vi "getConfigEventTest.vi"(8 "error in (no error)":errorcluster, 11 "SalProcess in":refnum<class "SalProcess.lvclass">) -> (0 "error out":errorcluster, 2 "configEventTest":cluster{"numOfTest":i32, "periodOfTestInMs":u32}, 3 "SalProcess out":refnum<class "SalProcess.lvclass">)   [LabVIEW 2018, in "SalProcess.lvclass"]
doc: "Get the configuration of event test."
uses:
  SalProcess.lvclass
  <vilib>/Utility/config.llb/Read Key (U32).vi
  <vilib>/Utility/config.llb/Read Key (I32).vi
  <vilib>/Utility/config.llb/NI_LVConfig.lvlib
panel:
  in  "configEventTestIn":cluster{"numOfTest":i32, "periodOfTestInMs":u32}
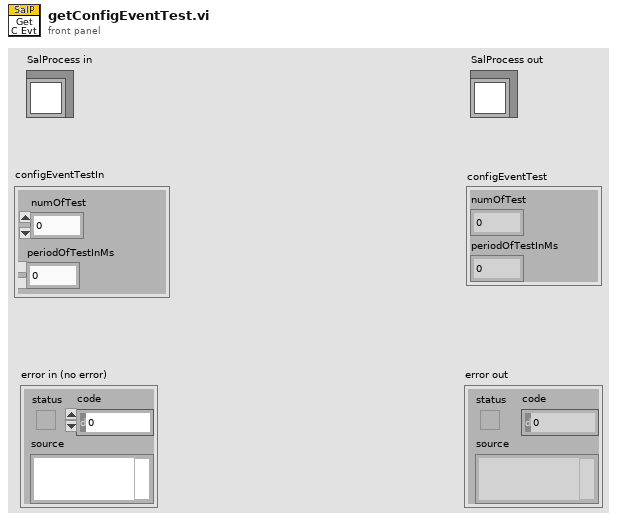
[diagram p1: front panel]
types:
  T1 = typedef "NI_LVConfig.lvlib/Config Data RefNum.ctl" = refnum<k1>
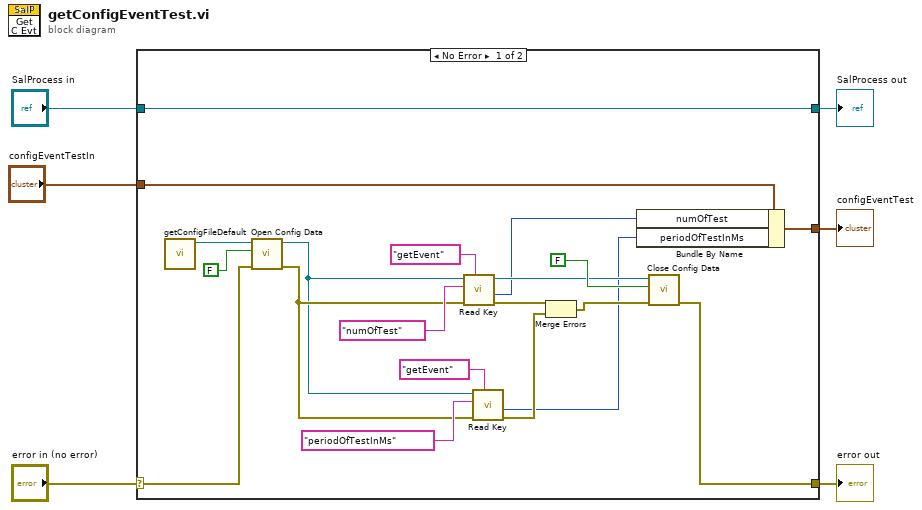
[diagram p0: block diagram]
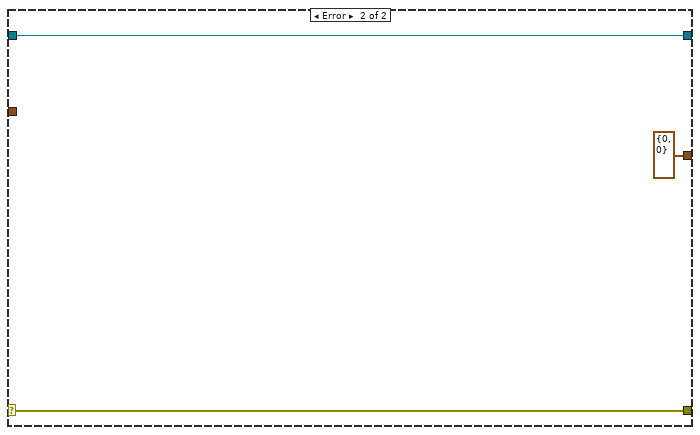
[diagram p2: hidden frame]
diagram:
  n1 = case shown="No Error" "error in (no error)" {
    selector: "error in (no error)" -> [w23 w29]
    tunnel: [w11 w29] -> w5
    tunnel: [w26 w28] -> w3
    tunnel: "SalProcess in" -> [w26 w28]
    tunnel: "configEventTestIn" -> [w10 _]
    tunnel: [w7 cluster{"numOfTest":i32, "periodOfTestInMs":i32} {"numOfTest"=0, "periodOfTestInMs"=0} ("configEventTest")] -> w1
    frame No Error {
      n2 = call "getConfigFileDefault.vi"() -> ("configFileDefault"=w25:path)  [unwired: 11 in]
      n3 = call <vilib>:"Open Config Data.vi"("error in (no error)"=w23, "create file if necessary (T)"=FALSE, "configuration file path"=w25) -> ("error out"=w16:errorcluster, "refnum"=w15:T1)  [unwired: 6 in, 1 out]
      n4 = call-poly <vilib>:"Read Key.vi"("section"="getEvent", "error in (no error)"=w16, "key"="numOfTest", "refnum"=w15) -> ("error out"=w14:errorcluster, "value"=w9:i32, "refnum out"=w19:T1)  [unwired: 4 in, 1 out]
      n5 = call-poly <vilib>:"Read Key.vi"("section"="getEvent", "error in (no error)"=w16, "key"="periodOfTestInMs", "refnum"=w15) -> ("error out"=w13:errorcluster, "value"=w8:u32)  [unwired: 4 in, 2 out]
      n6 = Merge Errors(w14, w13) -> (w12:errorcluster)
      n7 = Bundle By Name(cluster=w10, "numOfTest"=w9, "periodOfTestInMs"=w8) -> (w7:cluster{"numOfTest":i32, "periodOfTestInMs":u32})
      n8 = call <vilib>:"Close Config Data.vi"("error in (no error)"=w12, "write file if changed (T)"=FALSE, "refnum"=w19) -> ("error out"=w11:errorcluster)  [unwired: 7 in, 1 out]
    }
    frame Error {
    }
  }
  "error out" <- w5
  "SalProcess out" <- w3
  "configEventTest" <- w1
